vi "create CAD txt file.vi"() -> ()   [LabVIEW 2018]
panel:
  in  "radius (mm)":dbl
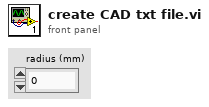
[diagram p1: front panel]
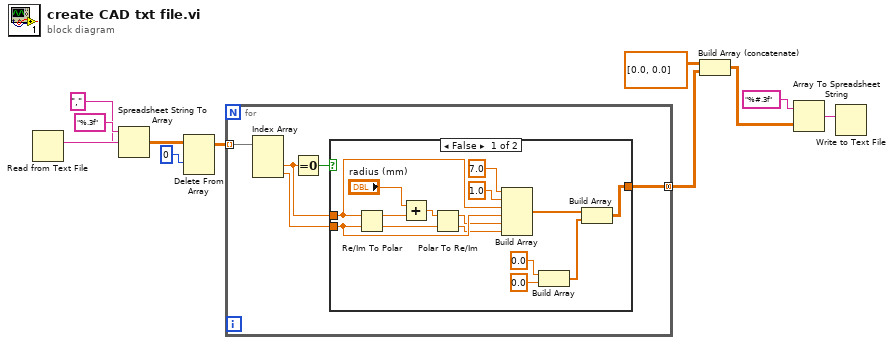
[diagram p0: block diagram]
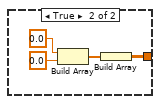
[diagram p2: hidden frame]
diagram:
  n1 = Read from Text File() -> (text=w11:string)  [unwired: 4 in, 3 out]
  n2 = Spreadsheet String To Array(delimiter (Tab)=",", format string="%.3f", spreadsheet string=w11) -> (array=w9:dbl[][])  [unwired: 1 in]
  n3 = Delete From Array(array=w9, index (row)=0) -> (array with subset deleted=w7:dbl[][])  [unwired: 2 in, 1 out]
  n4 = for {
    tunnel: w7 -> [w16] mode=indexing
    tunnel: [w14] -> w5 mode=concatenating
    n5 = Index Array(array=w16) -> (element #2=w12:dbl, element #3=w15:dbl)  [unwired: 3 in, 1 out]
    n6 = Equal To 0?(x=w12) -> (x = 0?=w13:bool)
    n7 = case shown="False" w13 {
      tunnel: w12 -> [w27 _]
      tunnel: w15 -> [w26 _]
      tunnel: [w17 w32] -> w14
      frame False {
        n8 = Re/Im To Polar(2:w26, 3:w27) -> (0:w28:dbl, 1:w31:dbl)
        n9 = Add(x="radius (mm)", y=w31) -> (x+y=w29:dbl)
        n10 = Polar To Re/Im(2:w28, 3:w29) -> (0:w24:dbl, 1:w25:dbl)
        n11 = Build Array(7.0 ("element"), 1.0 ("element"), w27, w26, w25, w24) -> (w19:dbl[])
        n12 = Build Array(0.0 ("element"), 0.0 ("element")) -> (w18:dbl[])
        n13 = Build Array(w19, w18) -> (w17:dbl[][])
      }
      frame True {
        n14 = Build Array(0.0 ("element"), 0.0 ("element")) -> (w33:dbl[])
        n15 = Build Array(w33) -> (w32:dbl[][])
      }
    }
  }
  n16 = Build Array (concatenate)(dbl[][] [[0.0, 0.0]] ("element"), w5) -> (w3:dbl[][])
  n17 = Array To Spreadsheet String(array=w3, 3:"%#.3f" ("format string")) -> (spreadsheet string=w2:string)  [unwired: 1 in]
  n18 = Write to Text File(text=w2) -> ()  [unwired: 3 in, 3 out]
